vi "Notifier_Driver.vi"(0 "Notification":bool, 2 "Notifier_Name":string, 11 "Error_In":errorcluster, 13 "Notifier_Operation_Select":T1=enum."Release_Notifier") -> (4 "Latest_Notification":bool, 15 "Error_Out":errorcluster)   [LabVIEW 2021]
doc: "Used to send the notification between loops"
uses:
  Controls/Notifier_Operation_Select.ctl
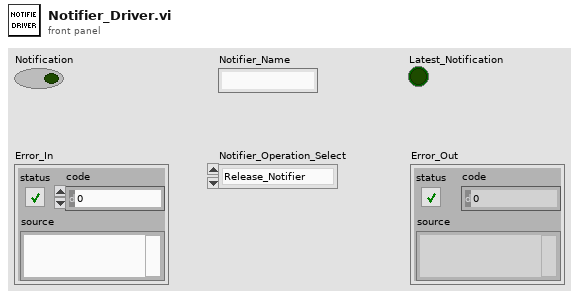
[diagram p1: front panel]
types:
  T1 = typedef "Notifier_Operation_Select.ctl" = enum16{"Obtain_Notifier", "Send_Notification", "Get_Notification_Status", "Release_Notifier"}
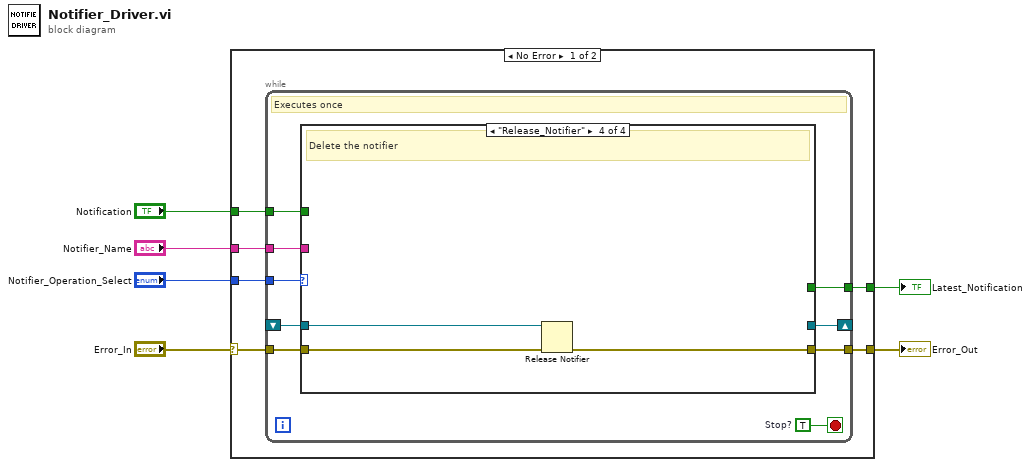
[diagram p0: block diagram]
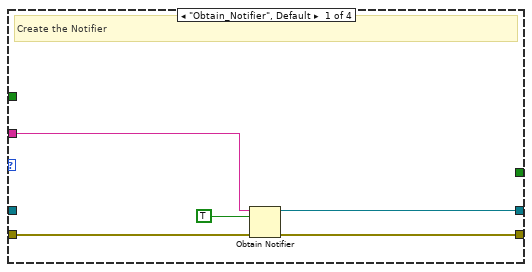
[diagram p2: hidden frame]
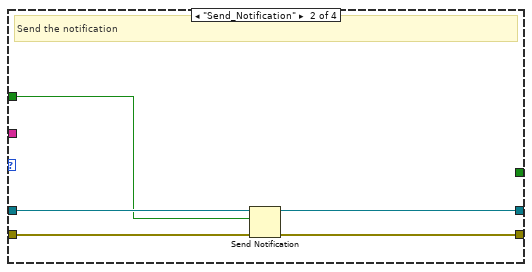
[diagram p3: hidden frame]
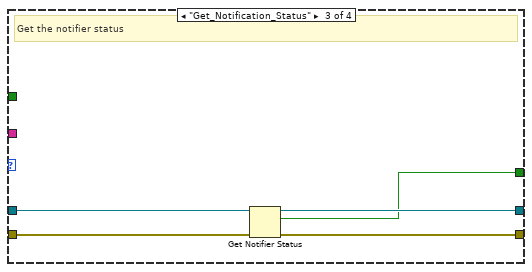
[diagram p4: hidden frame]
diagram:
  n1 = case shown="No Error" "Error_In" {
    selector: "Error_In" -> [w7 w40]
    tunnel: "Notifier_Operation_Select" -> [w12 _]
    tunnel: [w11 w40] -> w5
    tunnel: "Notifier_Name" -> [w10 _]
    tunnel: [w9 _] -> w3
    tunnel: "Notification" -> [w8 _]
    frame No Error {
      n2 = while {
        tunnel: w12 -> [w21]
        tunnel: w7 -> [w20]
        tunnel: [w19] -> w11
        shift-right: [w18] -> _
        shift-left: _ -> [w17]
        tunnel: w10 -> [w16]
        tunnel: [w15] -> w9
        tunnel: w8 -> [w13]
        stop <- w14 stop-if-true
        w14 = TRUE  # Stop?
        # "Executes once"
        n3 = case shown="\"Release_Notifier\"" w21 {
          tunnel: w20 -> [w26 w31 w36 w39]
          tunnel: [w25 w30 w35 w38] -> w19
          tunnel: [w22 w29 w33 _] -> w18
          tunnel: w17 -> [_ w28 w34 w37]
          tunnel: w16 -> [w24 _ _ _]
          tunnel: [_ _ w32 _] -> w15
          tunnel: w13 -> [_ w27 _ _]
          frame "Obtain_Notifier", Default {
            # "Create the Notifier"
            n4 = Obtain Notifier(name (unnamed)=w24, notification data type=TRUE, error in (no error)=w26) -> (notifier out=w22:refnum<notifier>, error out=w25:errorcluster)  [unwired: 1 in, 1 out]
          }
          frame "Send_Notification" {
            # "Send the notification"
            n5 = Send Notification(notification=w27, notifier=w28, error in (no error)=w31) -> (notifier out=w29:refnum<notifier>, error out=w30:errorcluster)
          }
          frame "Get_Notification_Status" {
            # "Get the notifier status"
            n6 = Get Notifier Status(notifier=w34, error in (no error)=w36) -> (notifier out=w33:refnum<notifier>, current notification=w32:bool, error out=w35:errorcluster)  [unwired: 2 out]
          }
          frame "Release_Notifier" {
            # "Delete the notifier"
            n7 = Release Notifier(notifier=w37, error in (no error)=w39) -> (error out=w38:errorcluster)  [unwired: 1 in, 2 out]
          }
        }
      }
    }
    frame Error {
    }
  }
  "Error_Out" <- w5
  "Latest_Notification" <- w3
